vi "DS345_BurstMode.get address.vi"(0 "i ref in":refnum<vi>, 5 "error in (no error)":errorcluster) -> (14 "i ref out":refnum<vi>, 16 "address":string, 19 "error out":errorcluster)   [LabVIEW 2014, in "DS345_BurstMode.lvlib"]
doc: "gets the GPIB address out of the BaseProcess i attributes. That string is needed when calling the instrument driver within the methods of this class."
uses:
  DS345_BurstMode.lvlib
  CS_Core/BaseProcess/BaseProcess.lvlib
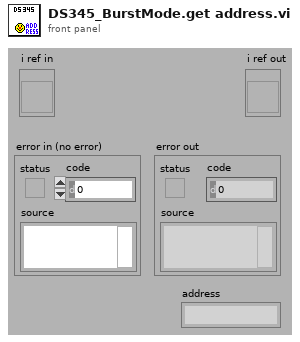
[diagram p1: front panel]
types:
  T1 = typedef "BaseProcess.lvlib/BaseProcess.i attribute.ctl" = cluster{"EventStatus":string, "EventError":i32, "PresetEvtWatchD":i32, "PresetPdcWatchD":i32, "EventTimeout":i32, "PeriodicInterval":i32, "Interface":string[], "Address":string[], "Special":string[], "PeriodicError":i32, "PeriodicStatus":string, "SuperProc":string, "Descriptors":T2[], "CaseRef":refnum<vi>, "PdcRef":refnum<vi>, "Thread Ref":refnum<vi>, "eventErrorID":i32, "eventStatusID":i32, "periodicErrorID":i32, "periodicStatusID":i32, "pdcCtrID":i32}
  T2 = typedef "BaseProcess.lvlib/BaseProcess.descriptor definition.ctl" = cluster{"selector":string, "descriptor":T3}
  T3 = typedef "BaseProcess.lvlib/BaseProcess.descriptor string definition.ctl" = string
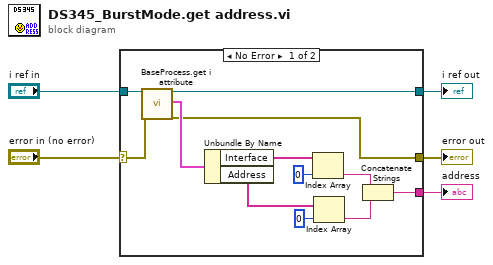
[diagram p0: block diagram]
diagram:
  n1 = case shown="No Error" "error in (no error)" {
    selector: "error in (no error)" -> [w6 w18]
    tunnel: "i ref in" -> [w17 w19]
    tunnel: [w9 _] -> w4
    tunnel: [w8 w19] -> w3
    tunnel: [w7 w18] -> w2
    frame No Error {
      n2 = call "BaseProcess.get i attribute.vi"("i ref in"=w17, "error in (no error)"=w6) -> ("i ref out"=w8:refnum<vi>, "i attribute"=w10:T1, "error out"=w7:errorcluster)  [unwired: 15 in]
      n3 = Unbundle By Name(w10) -> ("Interface"=w16:string[], "Address"=w13:string[])
      n4 = Index Array(array=w16, index=0 ("Index")) -> (element=w12:string)
      n5 = Index Array(array=w13, index=0 ("Index")) -> (element=w11:string)
      n6 = Concatenate Strings(w12, w11) -> (w9:string)
    }
    frame Error {
    }
  }
  "error out" <- w2
  "i ref out" <- w3
  "address" <- w4
